vi "得到label.vi"() -> ()   [LabVIEW 2015]
panel:
  in  "reference":refnum<vi>
  in  "Enum":enum16{"修改label位置", "讀取亂碼", "寫入正常"}(ring)=enum."讀取亂碼"
  in  "Data":string
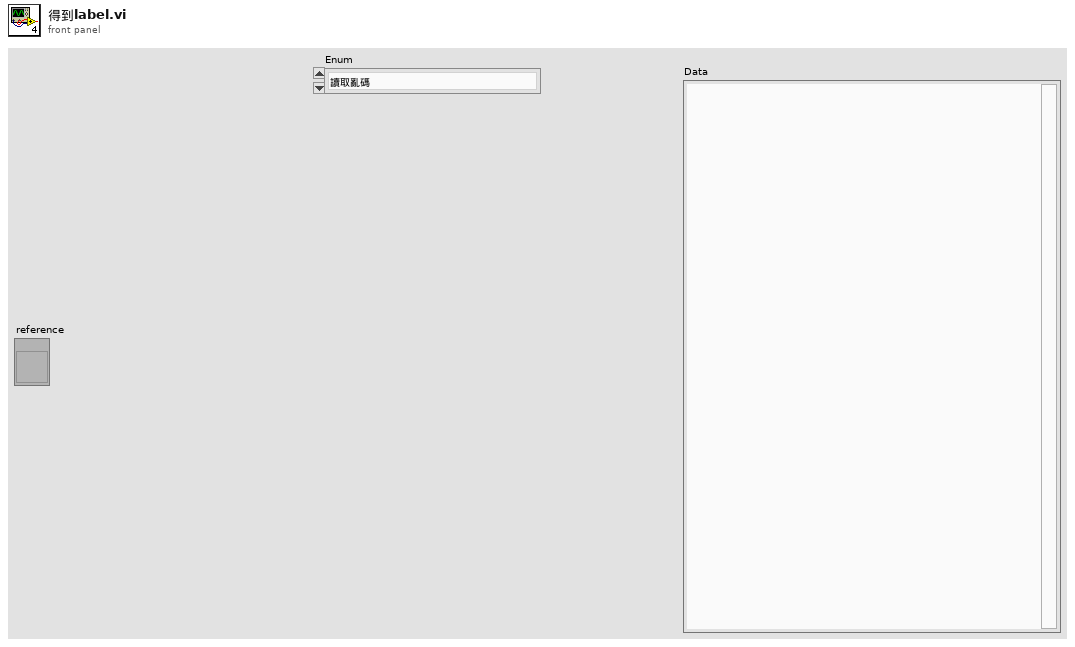
[diagram p1: front panel]
types:
  T1 = typedef "LVPositionTypeDef.ctl" = cluster{"Left":i32, "Top":i32}
  T2 = typedef "LVBoundsTypeDef.ctl" = cluster{"Width":u32, "Height":u32}
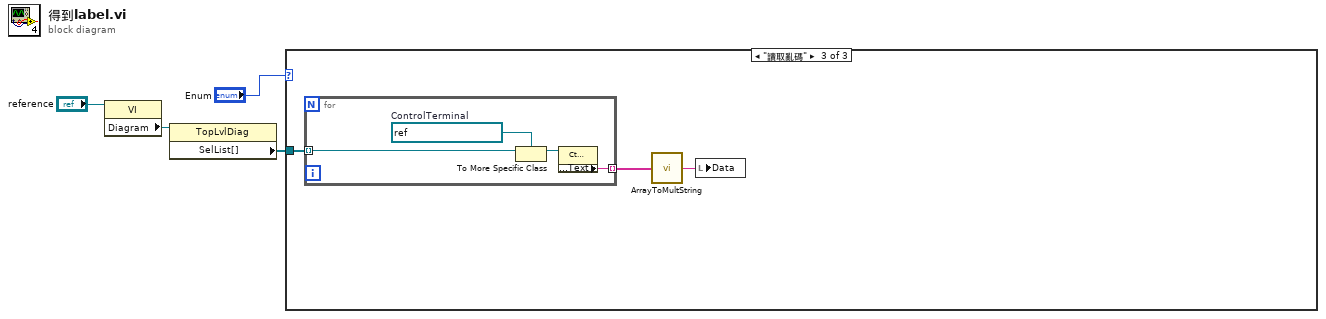
[diagram p0: block diagram]
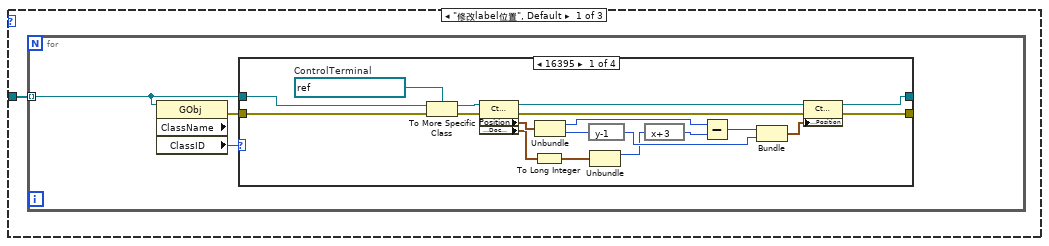
[diagram p2: hidden frame]
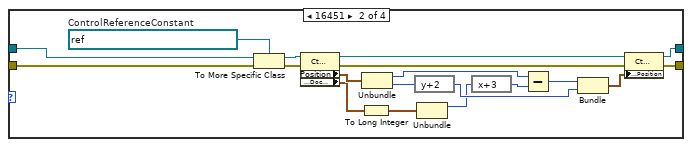
[diagram p3: hidden frame]
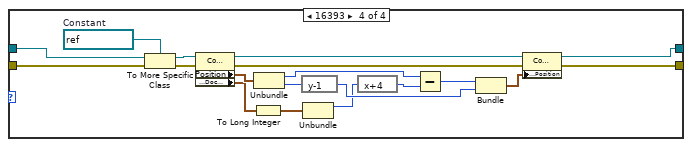
[diagram p5: hidden frame]
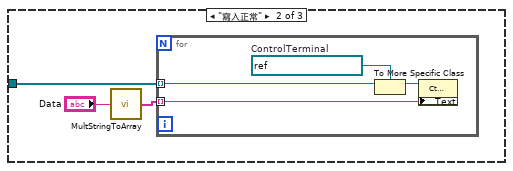
[diagram p6: hidden frame]
diagram:
  n1 = property class="VI"(reference="reference") -> ("Diagram"=w4:refnum<vi>)  [unwired: 1 in, 2 out]
  n2 = property class="TopLvlDiag"(reference=w4) -> ("SelList[]"=w3:refnum<vi>[])  [unwired: 1 in, 2 out]
  n3 = case shown="\"讀取亂碼\"" "Enum" {
    tunnel: w3 -> [w5 w69 w77]
    frame "修改label位置", Default {
      n4 = for {
        tunnel: w5 -> [w6] mode=indexing
        n5 = property on="Property Node" class="GObj" props=["ClassName", "ClassID"](reference=w6) -> (error out=w7:errorcluster, "ClassID"=w8:u32)  [unwired: 1 in, 2 out]
        n6 = case shown="16395" w8 {
          tunnel: w7 -> [w13 w46 w47 w51]
          tunnel: w6 -> [w14 w45 w48 w52]
          tunnel: [w12 w44 w48 w50] -> _
          tunnel: [w11 w43 w47 w49] -> _
          frame 16395 {
            w27 = refnum<vi> refnum  # ControlTerminal
            n7 = To More Specific Class(target class=w27, reference=w14, error in=w13) -> (specific class reference=w10:refnum<vi>, error out=w9:errorcluster)
            n8 = property on="Property Node" class="CtrlTerm"(reference=w10, error in=w9) -> (reference out=w26:refnum<vi>, error out=w17:errorcluster, "Position"=w25:T1, "Label.Doc Bounds"=w16:T2)
            n9 = To Long Integer(number=w16) -> (32bit integer=w15:cluster{"Width":i32, "Height":i32})
            n10 = Unbundle(w25) -> ("Left"=w20:i32, "Top"=w22:i32)
            n11 = expression code="y-1"(w22) -> (w23:i32)
            n12 = Unbundle(w15) -> ("Width"=w21:i32)  [unwired: 1 out]
            n13 = expression code="x+3"(w21) -> (w19:i32)
            n14 = Subtract(x=w20, y=w19) -> (x-y=w18:i32)
            n15 = Bundle(w18, "Top"=w23) -> (w24:cluster{i32, "Top":i32})  [unwired: 1 in]
            n16 = property on="Property Node" class="CtrlTerm"(reference=w26, error in=w17, "Label.Position"=w24) -> (reference out=w12:refnum<vi>, error out=w11:errorcluster)
          }
          frame 16451 {
            w42 = refnum<vi> refnum  # ControlReferenceConstant
            n17 = To More Specific Class(target class=w42, reference=w45, error in=w46) -> (specific class reference=w41:refnum<vi>, error out=w40:errorcluster)
            n18 = property on="Property Node" class="CtrlRefConst"(reference=w41, error in=w40) -> (reference out=w39:refnum<vi>, error out=w30:errorcluster, "Position"=w38:T1, "Label.Doc Bounds"=w29:T2)
            n19 = To Long Integer(number=w29) -> (32bit integer=w28:cluster{"Width":i32, "Height":i32})
            n20 = Unbundle(w38) -> ("Left"=w33:i32, "Top"=w35:i32)
            n21 = expression code="y+2"(w35) -> (w36:i32)
            n22 = Unbundle(w28) -> ("Width"=w34:i32)  [unwired: 1 out]
            n23 = expression code="x+3"(w34) -> (w32:i32)
            n24 = Subtract(x=w33, y=w32) -> (x-y=w31:i32)
            n25 = Bundle(w31, "Top"=w36) -> (w37:cluster{i32, "Top":i32})  [unwired: 1 in]
            n26 = property on="Property Node" class="CtrlRefConst"(reference=w39, error in=w30, "Label.Position"=w37) -> (reference out=w44:refnum<vi>, error out=w43:errorcluster)
          }
          frame Default {
          }
          frame 16393 {
            w67 = refnum<vi> refnum  # Constant
            n27 = To More Specific Class(target class=w67, reference=w52, error in=w51) -> (specific class reference=w66:refnum<vi>, error out=w65:errorcluster)
            n28 = property on="Property Node" class="Const"(reference=w66, error in=w65) -> (reference out=w64:refnum<vi>, error out=w55:errorcluster, "Position"=w63:T1, "Label.Doc Bounds"=w54:T2)
            n29 = To Long Integer(number=w54) -> (32bit integer=w53:cluster{"Width":i32, "Height":i32})
            n30 = Unbundle(w63) -> ("Left"=w58:i32, "Top"=w60:i32)
            n31 = expression code="y-1"(w60) -> (w61:i32)
            n32 = Unbundle(w53) -> ("Width"=w59:i32)  [unwired: 1 out]
            n33 = expression code="x+4"(w59) -> (w57:i32)
            n34 = Subtract(x=w58, y=w57) -> (x-y=w56:i32)
            n35 = Bundle(w56, "Top"=w61) -> (w62:cluster{i32, "Top":i32})  [unwired: 1 in]
            n36 = property on="Property Node" class="Const"(reference=w64, error in=w55, "Label.Position"=w62) -> (reference out=w50:refnum<vi>, error out=w49:errorcluster)
          }
        }
      }
    }
    frame "寫入正常" {
      n37 = call <userlib>:"MultStringToArray.vi"("String in"="Data") -> ("Array"=w70:string[])  [unwired: 14 in]
      n38 = for {
        tunnel: w69 -> [w74] mode=indexing
        tunnel: w70 -> [w71] mode=indexing
        w73 = refnum<vi> refnum  # ControlTerminal
        n39 = To More Specific Class(target class=w73, reference=w74) -> (specific class reference=w72:refnum<vi>)  [unwired: 1 in, 1 out]
        n40 = property class="CtrlTerm"(reference=w72, "Label.Text"=w71) -> ()  [unwired: 1 in, 2 out]
      }
    }
    frame "讀取亂碼" {
      n41 = for {
        tunnel: w77 -> [w80] mode=indexing
        tunnel: [w81] -> w76 mode=indexing
        w79 = refnum<vi> refnum  # ControlTerminal
        n42 = To More Specific Class(target class=w79, reference=w80) -> (specific class reference=w78:refnum<vi>)  [unwired: 1 in, 1 out]
        n43 = property class="CtrlTerm"(reference=w78) -> ("Label.Text"=w81:string)  [unwired: 1 in, 2 out]
      }
      n44 = call <userlib>:"ArrayToMultString.vi"("Value"=w76) -> ("Data"=w75:string)  [unwired: 14 in]
      n45 = local write "Data"(w75) -> ()
    }
  }
